vi "FT_Open_Device_By_Description.vi"(0 "Device Description":string) -> (1 "FT_Status":u32, 2 "Handle":u32)   [LabVIEW 2013]
uses:
  FTD2XX.dll
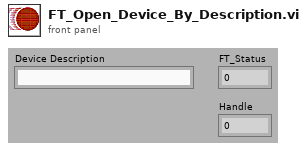
[diagram p1: front panel]
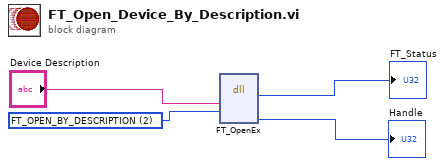
[diagram p0: block diagram]
diagram:
  w1 = u32 2 items=["FT_OPEN_BY_SERIAL_NUMBER"=1, "FT_OPEN_BY_DESCRIPTION"=2, "FT_OPEN_BY_LOCATION"=4] ("Flags")
  n1 = dll-call lib="FTD2XX.dll" fn="FT_OpenEx"("DeviceDescription"="Device Description", "Flags"=w1) -> ("FT_Status"=→"FT_Status":u32, "Handle"=→"Handle":u32)  [unwired: 6 in, 2 out]
